vi "Read Case Selector.vi"(8 "error in (no error)":errorcluster, 11 "Case Structure in":refnum<class "Case Structure.lvclass">) -> (0 "error out":errorcluster, 2 "Tunnel":T1, 3 "Case Structure out":refnum<class "Case Structure.lvclass">)   [LabVIEW 2025, in "Case Structure.lvclass"]
uses:
  Case Structure.lvclass
  Controls/Tunnel.ctl
  Controls/Terminal.ctl
  Controls/wire.ctl
  Case Structure.lvclass/Case Structure.ctl
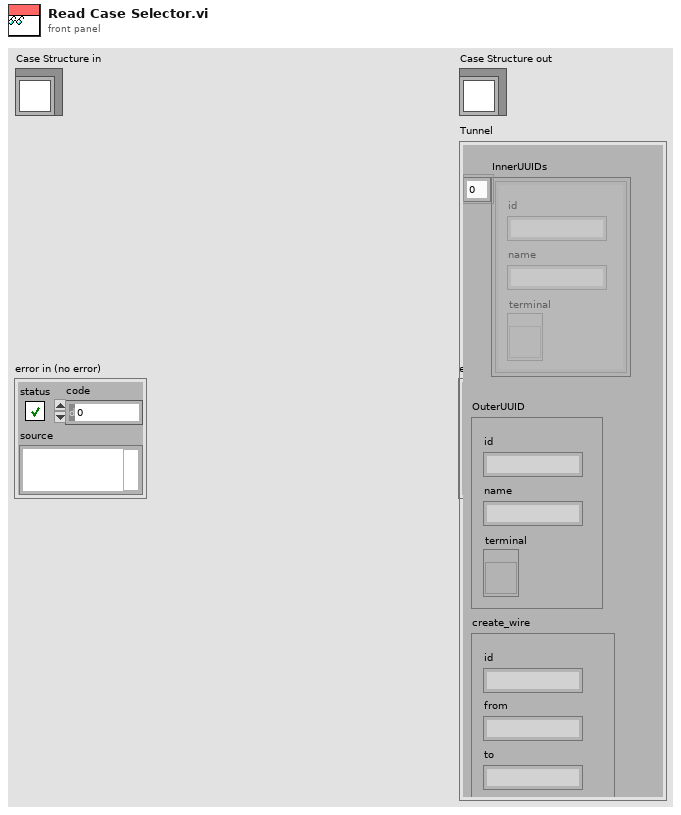
[diagram p1: front panel]
types:
  T1 = typedef "Tunnel.ctl" = cluster{"OuterUUID":T2, "InnerUUIDs":T2[], "create_wire":T3}
  T2 = typedef "Terminal.ctl" = cluster{"id":string, "name":string, "terminal":refnum<vi>}
  T3 = typedef "wire.ctl" = cluster{"id":string, "from":string, "to":string}
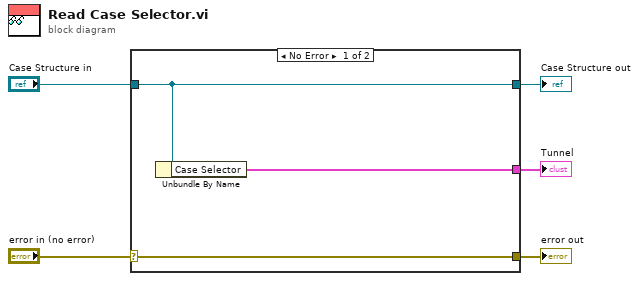
[diagram p0: block diagram]
diagram:
  n1 = case shown="No Error" "error in (no error)" {
    selector: "error in (no error)" -> [w8 w9]
    tunnel: [w8 w9] -> w4
    tunnel: [w7 w10] -> w2
    tunnel: "Case Structure in" -> [w7 w10]
    tunnel: [w6 _] -> w1
    frame No Error {
      n2 = Unbundle By Name(w7) -> ("Case Selector"=w6:T1)
    }
    frame Error {
    }
  }
  "error out" <- w4
  "Case Structure out" <- w2
  "Tunnel" <- w1
